vi "OpenPort.vi"(1 "Port":refnum<visa-resource-name>) -> (0 "Serial port":refnum<visa-resource-name>)   [LabVIEW 2021]
uses:
  <vilib>/Instr/_visa.llb/VISA Configure Serial Port (Instr).vi
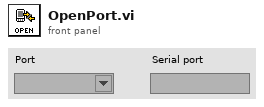
[diagram p1: front panel]
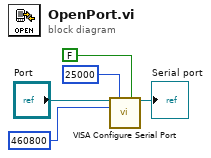
[diagram p0: block diagram]
diagram:
  n1 = call-poly "VISA Configure Serial Port"("VISA resource name"="Port", "timeout (10sec)"=u32 25000, "Enable Termination\nChar (T)"=FALSE ("Enable Termination\nChar (T)"), "baud rate (9600)"=u32 460800) -> ("VISA resource name out"=→"Serial port":refnum<visa-resource-name>)  [unwired: 10 in, 1 out]
